vi "Control - PID Control.vi"() -> ()   [LabVIEW 2013, in "PID Control Workspace Object.lvlib"]
doc: "Sample numeric display item."
uses:
  PID Control Workspace Object.lvlib
  <vilib>/NI Veristand/Display Template Support/Display Template Support.llb/cluster_Screen Item Settings.ctl
  <vilib>/NI Veristand/Display Template Support/Display Template Support.llb/cluster_Graph Scale Settings.ctl
  <vilib>/NI Veristand/Display Template Support/Display Template Support.llb/cluster_Graph Plot Settings.ctl
  NationalInstruments.VeriStand.SystemStorage
  <vilib>/NI Veristand/Display Template Support/Display Template Support.llb/enum_Display Template Handler Minimal To Widget Msg.ctl
  <vilib>/NI Veristand/Display Template Support/Display Template Support.llb/enum_Display Template Handler Minimal To Workspace.ctl
  Shared/Types/Workspace Object Cached Settings.ctl
  Shared/Types/Workspace Object State Variables.ctl
  <vilib>/NI Veristand/Execution/Workspace/UDPChannelStreamSession.ctl
  Shared/Types/UDP Streaming Command Cluster.ctl
  Shared/Types/UDP Streaming State.ctl
  NationalInstruments.VeriStand.ClientAPI
  <vilib>/NI Veristand/Execution/Workspace/UDP Stream Packet.ctl
  <vilib>/NI Veristand/Display Template Support/Display Template Support.llb/sub_Display Template Handler Custom.vi
  Shared/Constants.vi
  <vilib>/NI Veristand/Execution/Workspace/NI VeriStand - Set Single Channel Value.vi
  <vilib>/NI Veristand/Execution/Workspace/NI VeriStand - Get Multiple Channel Values.vi
  <vilib>/Utility/tcp.llb/UDP Multicast Read-Only Open.vi
  Shared/Control Addon Shared.lvlib
  <vilib>/NI Veristand/Execution/Workspace/NI_VS Workspace ExecutionAPI.lvlib
panel:
  in  "Revert":bool
  in  "Apply":bool
  in  "Manual Output":dbl
  in  "Manual Control":bool
  in  "Setpoint":dbl
  in  "NIVS.System Definition Root":refnum<k24>
  in  "NIVS.Gateway IP Address":string
  in  "Hold":bool
  in  "Autoscale Y":bool=TRUE
  in  "Autoscale X":bool=TRUE
  out "Chart":waveform(dbl)[](graph)
  out "Control Name":string
  in  "Item.Data":T1
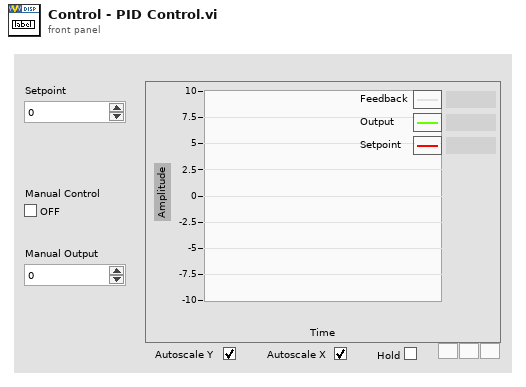
[diagram p1: front panel]
types:
  T1 = typedef "cluster_Screen Item Settings.ctl" = cluster{"Template VI":string, "Position X":i32, "Position Y":i32, "Custom":string, "Show Title Bar":bool, "ID":i32, "Always On Top":bool, "Allow Resize":bool, "Allow Minimize":bool, "Allow Close":bool, "Size to Screen":bool, "Screen.ID":i32, "State":enum16{"Normal", "New"}, "Title":string, "Window Bounds":cluster{"[0]":i16, "[1]":i16, "[2]":i16, "[3]":i16}, "Channel Ref":u64, "Unit":string, "Default Units?":bool, "Flash Limit?":bool, "Color 1":u32, "Color 2":u32, "Color 3":u32, "Color 4":u32, "Bck Color":u32, "Fore Color":u32, "Limit 1":dbl, "Limit 2":dbl, "Limit 3":dbl, "Limit 4":dbl, "Limit Mode 1":i32, "Limit Mode 2":i32, "Limit Mode 3":i32, "Limit Mode 4":i32, "Scale Precision":i32, "Scale Min":dbl, "Scale Max":dbl, "Format":i32, "Precision":i32, "Background Type":i32, "IDs":i32[], "Units":string[], "Labels":string[], "Scale Factor":dbl, "Scale Offset":dbl, "YScale Index":u32[], "XScale":T2, "YScales":T2[], "Plots":T3[], "Update Period":dbl, "History Length":dbl, "My.Ref":refnum<vi>, "Is Control?":bool, "Channel Paths":string[], "Custom Data":variant}
  T2 = typedef "cluster_Graph Scale Settings.ctl" = cluster{"Format":u8, "Precision":u8, "Fit":u8, "Label":string, "Use Default Label":bool, "Label Visible":bool, "Min":dbl, "Max":dbl}
  T3 = typedef "cluster_Graph Plot Settings.ctl" = cluster{"Bar Style":u8, "Fill To":i16, "Fill/PtColor":u32, "Line Style":u8, "Line Width":u8, "Color":u32, "Interp":u8, "Point Style":u8}
  T4 = typedef "Control Addon Shared.lvlib/UDP Streaming State.ctl" = enum8{"Idle", "Start Acq", "Run", "Stop Acq", "Exit"}
  T5 = typedef "Control Addon Shared.lvlib/UDP Streaming Command Cluster.ctl" = cluster{"Action":T4, "Channels":string[]}
  T6 = typedef "NI_VS Workspace ExecutionAPI.lvlib/UDPChannelStreamSession.ctl" = refnum<k24>
  T7 = cluster{"Initialized Waveform":waveform(dbl)[], "VS UDP Session":T6, "Channel IDs":i32[], "Packet IDs":i32[], "Max Packet Size":i32, "UDP Ref":refnum<k16>}
  T8 = typedef "Control Addon Shared.lvlib/Workspace Object State Variables.ctl" = cluster{"Cached":T9, "Found?":bool, "UDP Channels":string[], "Connected?":bool, "Previous Values":dbl[], "Slow Channels":string[], "Pending Change?":bool}
  T9 = typedef "Control Addon Shared.lvlib/Workspace Object Cached Settings.ctl" = cluster{"Path":string}
  T10 = typedef "enum_Display Template Handler Minimal To Workspace.ctl" = cluster{"Operation":enum16{"SetCustomData", "DeleteItem"}, "Data":variant}
  T11 = typedef "enum_Display Template Handler Minimal To Widget Msg.ctl" = enum16{"Stop", "LaunchConfigDialog"}
  T12 = typedef "NI_VS Workspace ExecutionAPI.lvlib/WorkspaceAPI.ctl" = refnum<k24>
  T13 = typedef "NI_VS Workspace ExecutionAPI.lvlib/SystemStateEventRef.ctl" = cluster{"CustDatRef":refnum<user-event>, "EvtRef":refnum<k27>}
  T14 = typedef "NI_VS Workspace ExecutionAPI.lvlib/SystemStateRegEventRef.ctl" = refnum<event-registration>
  T15 = cluster{"Event Registration Refnum":refnum<event-registration>, "SystemChangeEventRef":T14}
  T16 = typedef "NI_VS Workspace ExecutionAPI.lvlib/SystemState.ctl" = u8
  T17 = typedef "NI_VS Workspace ExecutionAPI.lvlib/UDP Stream Packet.ctl" = cluster{"ID":i32, "t0":dbl, "dt":dbl, "Channel IDs":i32[], "Channel Data":dbl[][], "Sample Offset":u64}
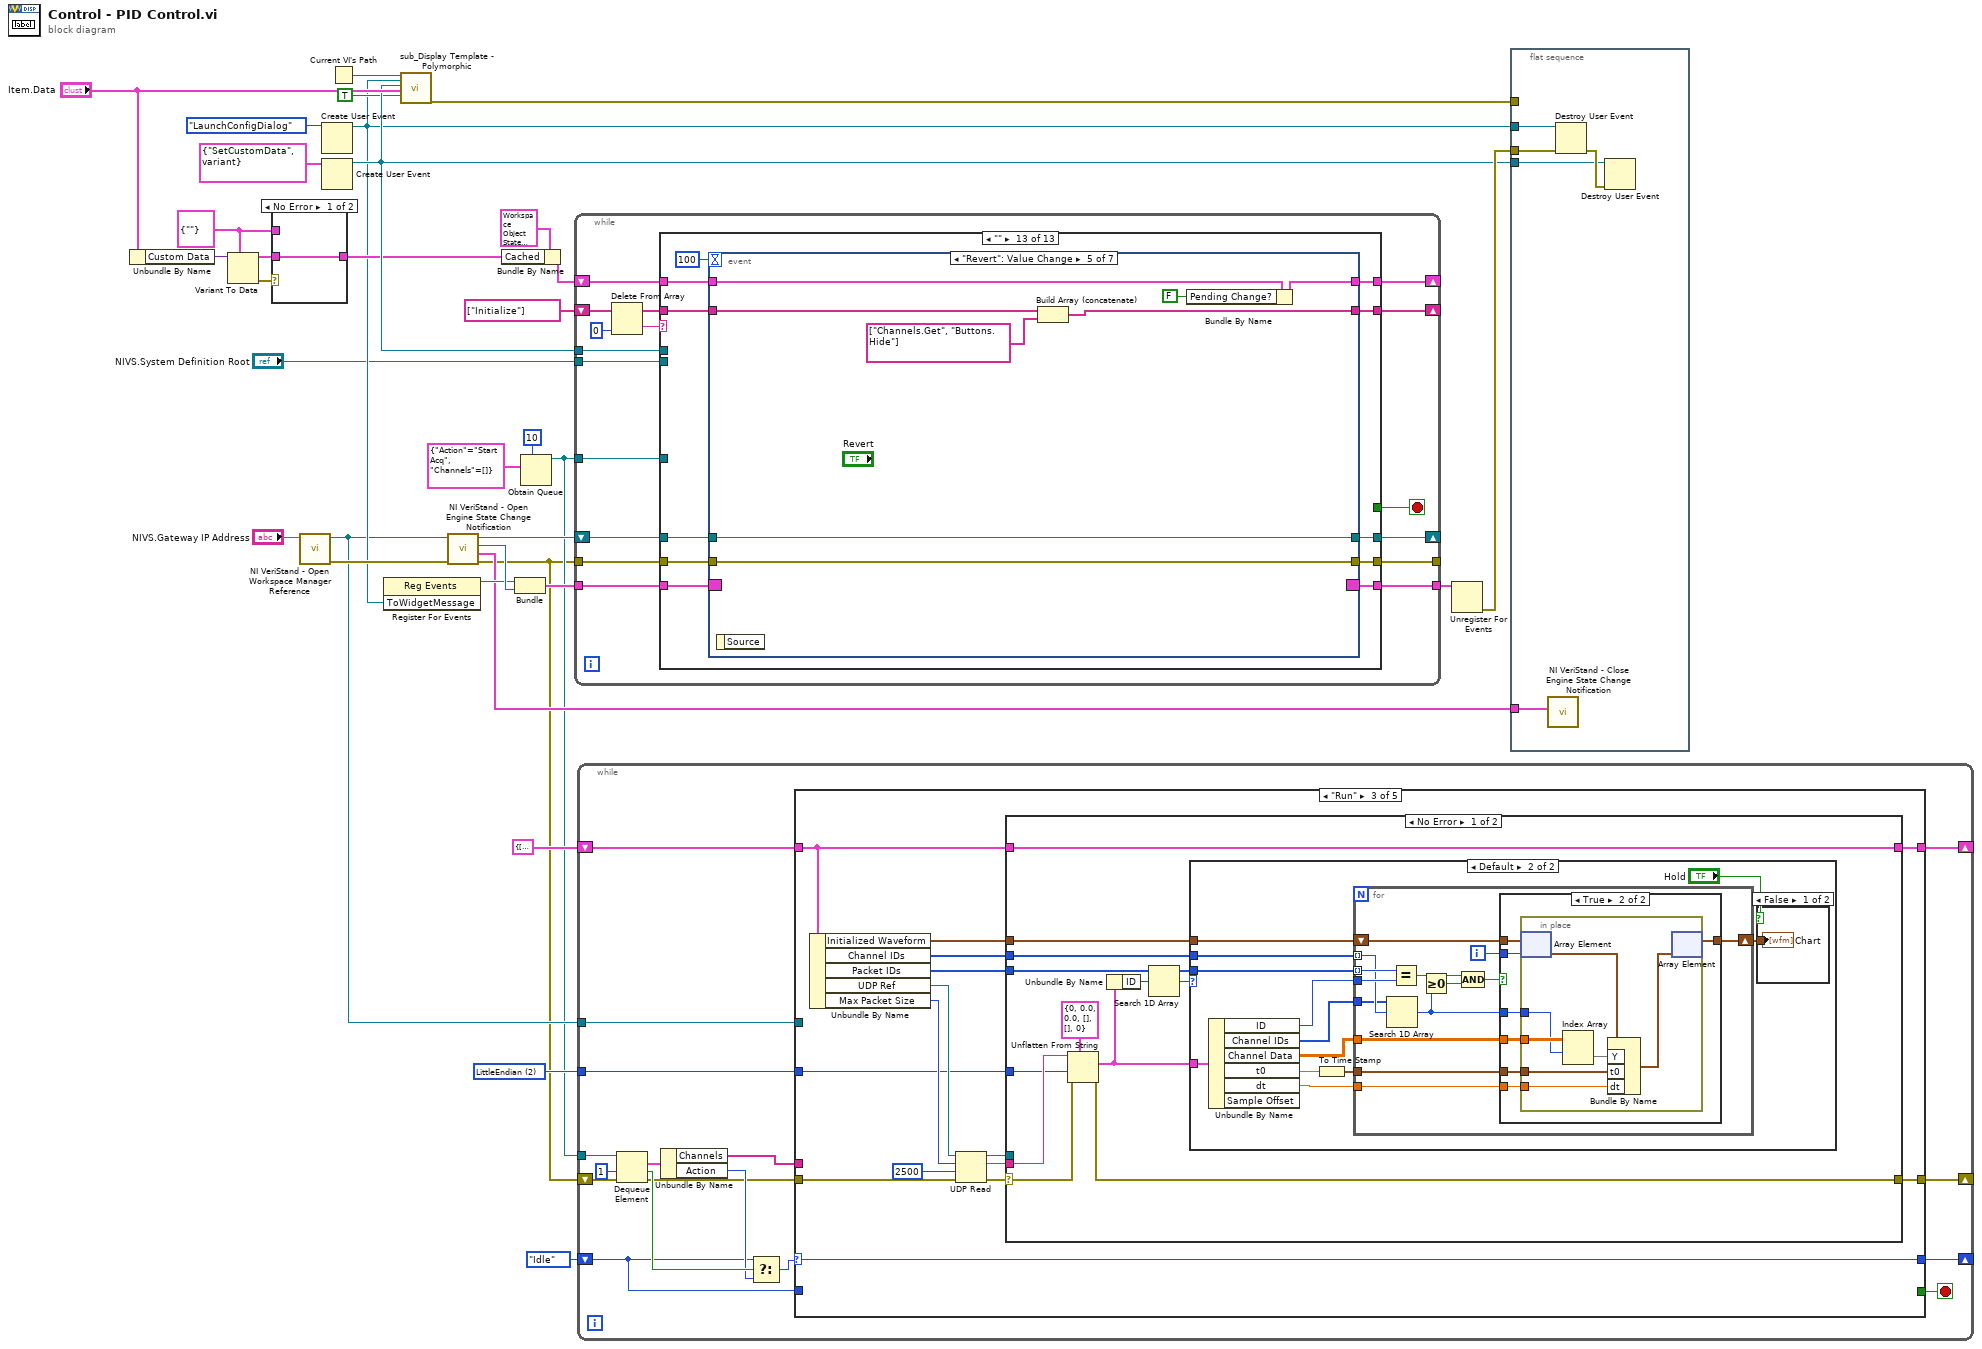
[diagram p0: block diagram]
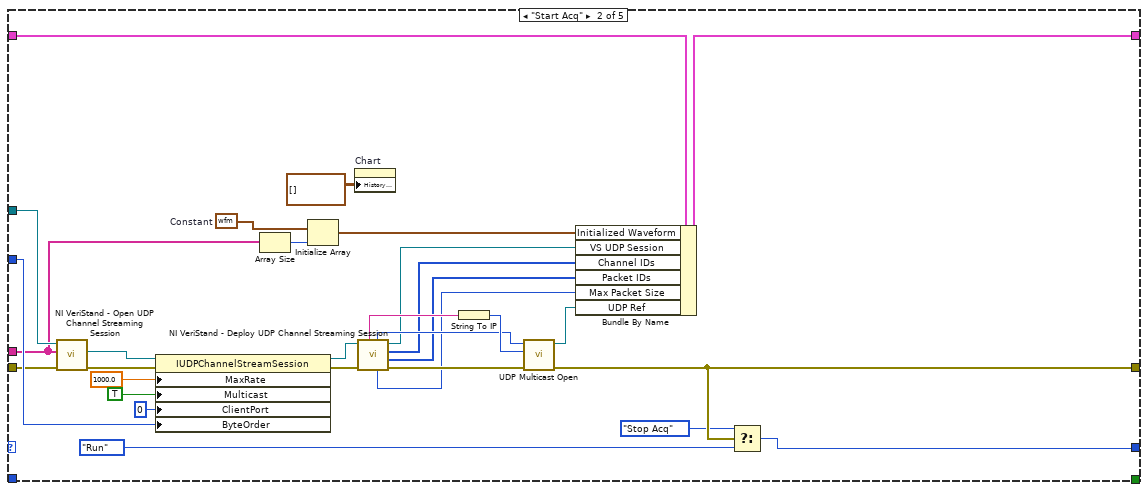
[diagram p3: hidden frame]
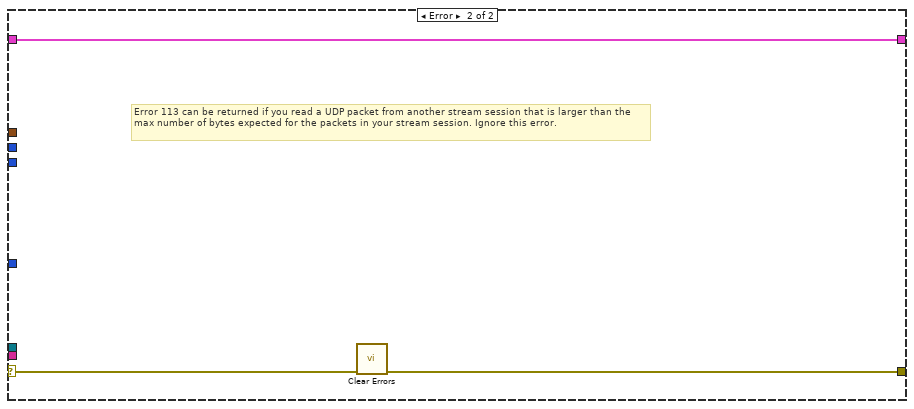
[diagram p7: hidden frame]
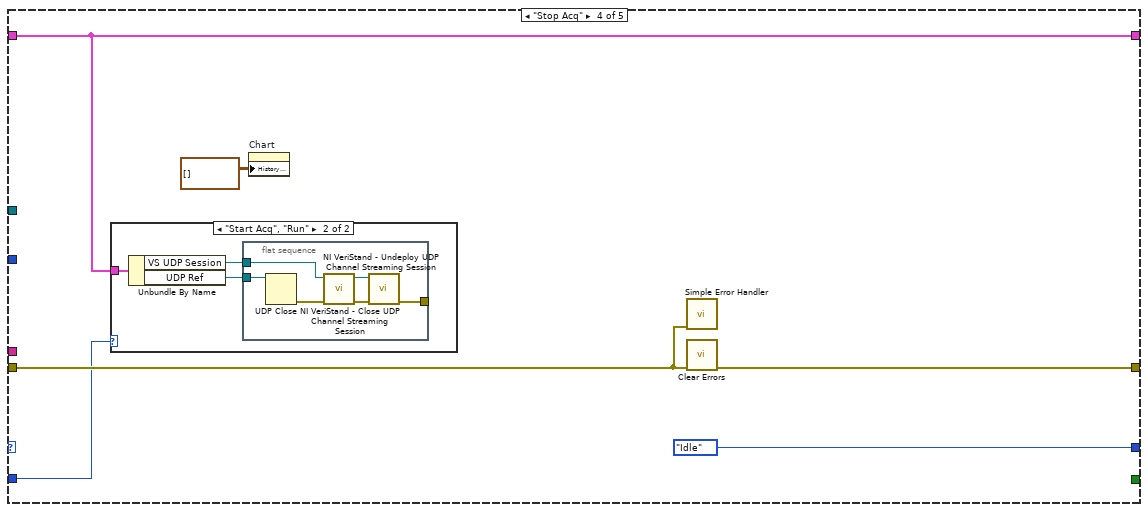
[diagram p8: hidden frame]
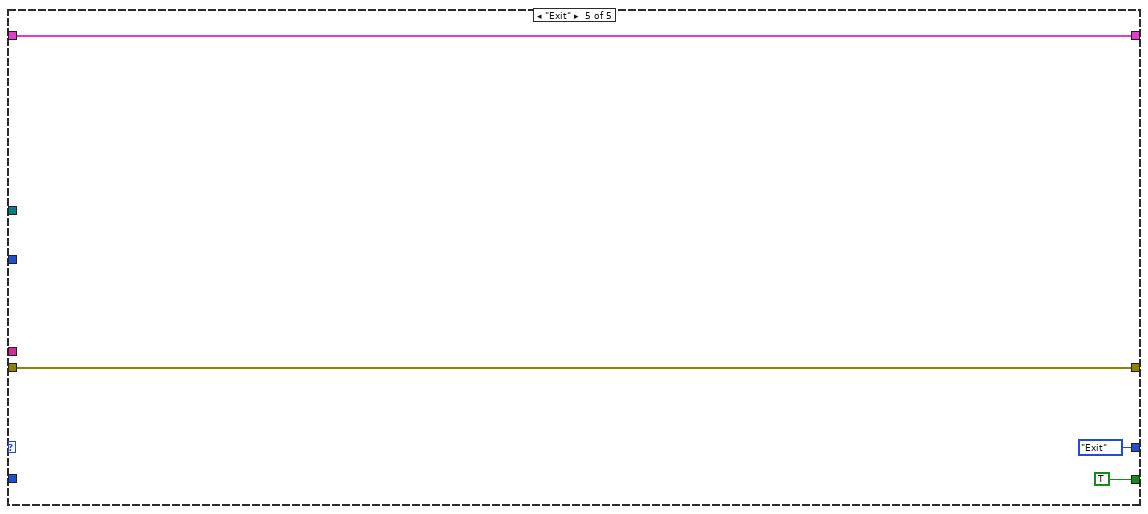
[diagram p10: hidden frame]
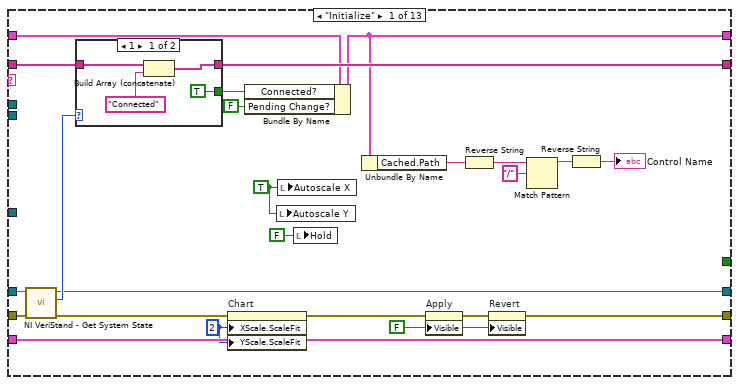
[diagram p12: hidden frame]
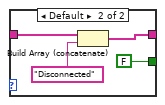
[diagram p13: hidden frame]
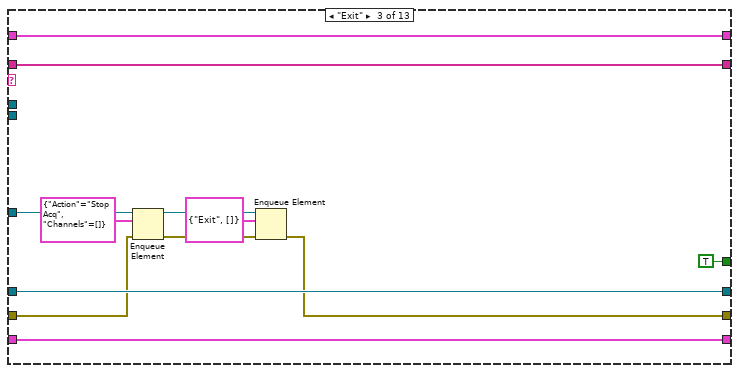
[diagram p15: hidden frame]
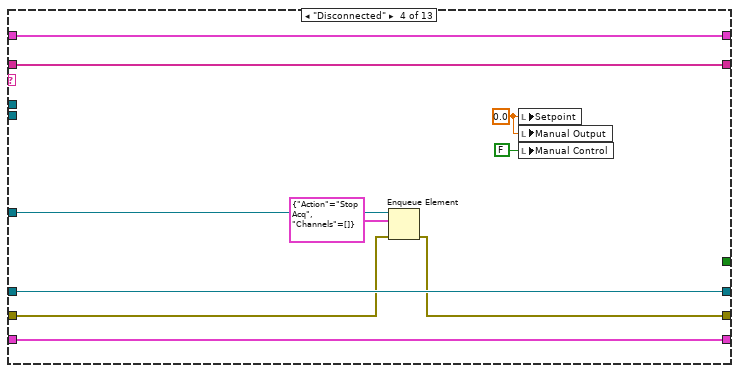
[diagram p16: hidden frame]
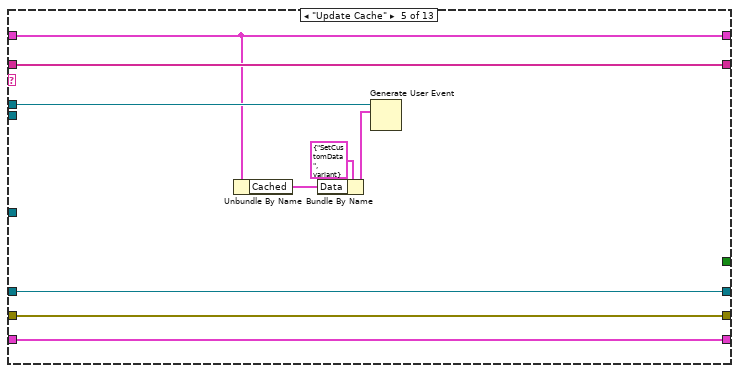
[diagram p17: hidden frame]
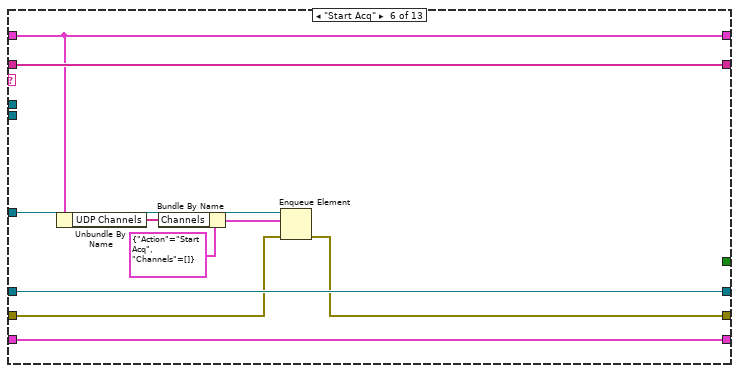
[diagram p18: hidden frame]
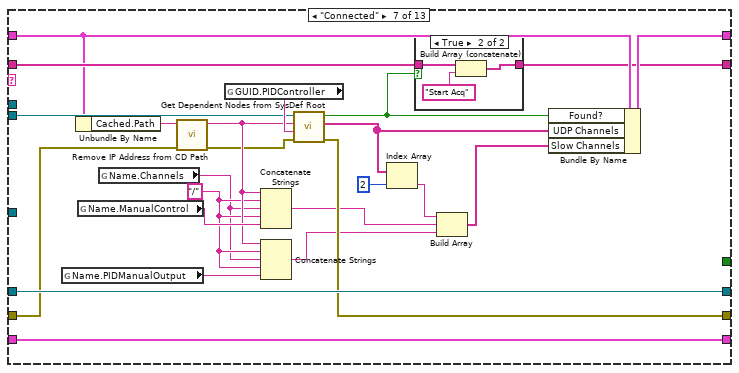
[diagram p19: hidden frame]
diagram:
  w6 = 2 items=["BigEndian", "NativeHostOrder", "LittleEndian"] ("Byte Order")
  w14 = T9 {"Path"=""}
  n1 = Unbundle By Name("Item.Data") -> ("Custom Data"=w18:variant)
  n2 = Variant To Data(type=w14, Variant=w18) -> (data=w15:T9, error out=w16:errorcluster)  [unwired: 1 in]
  n3 = case shown="No Error" w16 {
    tunnel: w15 -> [w35 _]
    tunnel: [w35 w36] -> w11
    tunnel: w14 -> [_ w36]
    frame No Error {
    }
    frame Error {
    }
  }
  n4 = call <vilib>:"NI VeriStand - Open Workspace Manager Reference.vi"("Gateway IP Address (\"\": localhost)"="NIVS.Gateway IP Address") -> ("error out"=w25:errorcluster, "WorkspaceManager"=w8:T12)  [unwired: 9 in]
  n5 = Create User Event(user event datatype=enum_Display_Template_Handler_Minimal_To_Widget_Msg."LaunchConfigDialog" ("ToWidgetMessage")) -> (user event=w10:refnum<user-event>)  [unwired: 1 in, 1 out]
  n6 = Create User Event(user event datatype=T10 {"Operation"=enum."SetCustomData", "Data"=variant} ("Data")) -> (user event=w28:refnum<user-event>)  [unwired: 1 in, 1 out]
  n7 = Current VI's Path() -> (path=w30:path)
  n8 = register-events(w10) -> (reference out=w23:refnum<event-registration>)  [unwired: 2 in, 1 out]
  n9 = call-poly <vilib>:"sub_Display Template - Polymorphic.vi"("Parent.Path"=w30, "ToWidgetEvent"=w10, "ToWorkspace"=w28, "Item.Data"="Item.Data", "Resizable"=TRUE) -> ("error out"=w34:errorcluster)  [unwired: 1 in, 13 out]
  n10 = call <vilib>:"NI VeriStand - Open Engine State Change Notification.vi"("error in (no error)"=w25, "WorkspaceManager in"=w8) -> ("error out"=w1:errorcluster, "SystemStateRefs"=w21:T13, "SystemChangeEventRef"=w24:T14, "WorkspaceManager out"=w19:T12)  [unwired: 6 in]
  n11 = Bundle By Name(cluster=T8 {"Cached"={"Path"=""}, "Found?"=FALSE, "UDP Channels"=[], "Connected?"=FALSE, "Previous Values"=[0.0, 0.0, 0.0], "Slow Channels"=[], "Pending Change?"=FALSE}, "Cached"=w11) -> (w12:T8)
  n12 = Bundle("Event Registration Refnum"=w23, "SystemChangeEventRef"=w24) -> (w22:T15)  [unwired: 1 in]
  n13 = Obtain Queue(max queue size (-1, unlimited)=10, element data type=T5 {"Action"=enum."Start Acq", "Channels"=[]}) -> (queue out=w3:refnum<queue>)  [unwired: 3 in, 2 out]
  n14 = while {
    tunnel: w22 -> [w53]
    tunnel: w28 -> [w51]
    shift-right: [w45] -> _
    shift-left: string[] ["Initialize"] -> [w49]
    shift-right: [w43] -> _
    shift-left: w19 -> [w42]
    tunnel: w1 -> [w47]
    tunnel: [w44] -> w17
    tunnel: [w40] -> _
    shift-right: [w39] -> _
    shift-left: w12 -> [w41]
    tunnel: "NIVS.System Definition Root" -> [w38]
    tunnel: w3 -> [w37]
    stop <- w52 stop-if-true
    n15 = Delete From Array(array=w49, index=0) -> (deleted portion=w48:string, array with subset deleted=w46:string[])  [unwired: 1 in]
    n16 = case shown="\"\"" w48 {
      tunnel: w53 -> [w71 w89 w101 w111 w120 w130 w154 w171 w198 w230 w238 w256 w277]
      tunnel: [_ _ TRUE _ _ _ _ _ _ _ _ _ _] -> w52
      tunnel: [w73 w90 w102 w112 w121 w131 w137 w161 w199 w231 w239 w257 w274] -> w45
      tunnel: w51 -> [_ _ _ _ w117 _ _ _ _ _ _ _ _]
      tunnel: w47 -> [w76 w87 w93 w107 w118 w123 w141 w169 w186 w225 w233 w244 w270]
      tunnel: w46 -> [w74 w90 w102 w112 w121 w131 w155 w160 w199 w231 w239 w257 w273]
      tunnel: [w71 w89 w101 w111 w120 w130 w154 w171 w198 w230 w238 w256 w275] -> w44
      tunnel: [w72 w88 w100 w110 w119 w129 w153 w170 w183 w229 w237 w242 w271] -> w43
      tunnel: w42 -> [w75 w88 w100 w110 w119 w129 w153 w170 w184 w229 w237 w245 w272]
      tunnel: w41 -> [w65 w86 w99 w109 w114 w128 w149 w165 w182 w228 w236 w240 w267]
      tunnel: [w55 w87 w92 w106 w118 w122 w152 w169 w185 w224 w232 w243 w269] -> w40
      tunnel: [w64 w86 w99 w109 w114 w128 w148 w164 w181 w228 w236 w241 w268] -> w39
      tunnel: w38 -> [_ _ _ _ _ _ w150 w167 _ _ _ _ _]
      tunnel: w37 -> [_ _ w98 w108 _ w127 _ _ _ _ _ _ _]
      frame "Initialize" {
        w54 = FALSE ("Hold")
        w61 = u8 2 ("X Scale.Scale Fit")
        w62 = TRUE ("Autoscale X")
        n17 = call <vilib>:"NI VeriStand - Get System State.vi"("error in (no error)"=w76, "WorkspaceManager in"=w75) -> ("error out"=w60:errorcluster, "System State"=w77:T16, "WorkspaceManager  out"=w72:T12)  [unwired: 5 in, 2 out]
        n18 = case shown="1" w77 {
          tunnel: w74 -> [w81 w85]
          tunnel: [w80 w84] -> w73
          tunnel: [TRUE FALSE] -> w63
          frame 1 {
            n19 = Build Array (concatenate)(w81, "Connected") -> (w80:string[])
          }
          frame Default {
            n20 = Build Array (concatenate)(w85, "Disconnected") -> (w84:string[])
          }
        }
        n21 = property on="Chart" class="WFChart (strict)"(error in=w60, "XScale.ScaleFit"=w61, "YScale.ScaleFit"=w61) -> (error out=w57:errorcluster)  [unwired: 1 in, 1 out]
        n22 = Bundle By Name(cluster=w65, "Connected?"=w63, "Pending Change?"=FALSE) -> (w64:T8)
        n23 = local write "Autoscale Y"(w62) -> ()
        n24 = local write "Autoscale X"(w62) -> ()
        n25 = local write "Hold"(FALSE ("Hold")) -> ()
        n26 = Unbundle By Name(w64) -> ("Cached.Path"=w67:string)
        n27 = property on="Apply" class="Bool"(error in=w57, "Visible"=w54) -> (error out=w56:errorcluster)  [unwired: 1 in, 1 out]
        n28 = Reverse String(1:w67) -> (0:w70:string)
        n29 = property on="Revert" class="Bool"(error in=w56, "Visible"=w54) -> (error out=w55:errorcluster)  [unwired: 1 in, 1 out]
        n30 = Match Pattern(string=w70, regular expression="/") -> (before substring=w66:string)  [unwired: 1 in, 3 out]
        n31 = Reverse String(1:w66) -> (0:→"Control Name":string)
      }
      frame Default {
      }
      frame "Exit" {
        n32 = Enqueue Element(queue=w98, element=T5 {"Action"=enum."Stop Acq", "Channels"=[]}, error in (no error)=w93) -> (queue out=w96:refnum<queue>, error out=w94:errorcluster)  [unwired: 1 in, 1 out]
        n33 = Enqueue Element(queue=w96, element=T5 {"Action"=enum."Exit", "Channels"=[]}, error in (no error)=w94) -> (error out=w92:errorcluster)  [unwired: 1 in, 2 out]
      }
      frame "Disconnected" {
        w104 = 0.0 ("Setpoint")
        n34 = Enqueue Element(queue=w108, element=T5 {"Action"=enum."Stop Acq", "Channels"=[]}, error in (no error)=w107) -> (error out=w106:errorcluster)  [unwired: 1 in, 2 out]
        n35 = local write "Setpoint"(w104) -> ()
        n36 = local write "Manual Output"(w104) -> ()
        n37 = local write "Manual Control"(FALSE ("Manual Control")) -> ()
      }
      frame "Update Cache" {
        n38 = Unbundle By Name(w114) -> ("Cached"=w113:T9)
        n39 = Bundle By Name(cluster=T10 {"Operation"=enum."SetCustomData", "Data"=variant} ("event data"), "Data"=w113) -> (w115:T10)
        n40 = Generate User Event(user event=w117, event data cluster=w115) -> ()  [unwired: 2 in, 2 out]
      }
      frame "Start Acq" {
        n41 = Unbundle By Name(w128) -> ("UDP Channels"=w125:string[])
        n42 = Bundle By Name(cluster=T5 {"Action"=enum."Start Acq", "Channels"=[]}, "Channels"=w125) -> (w124:T5)
        n43 = Enqueue Element(queue=w127, element=w124, error in (no error)=w123) -> (error out=w122:errorcluster)  [unwired: 1 in, 2 out]
      }
      frame "Connected" {
        w134 = "/" ("string")
        n44 = global read "Constants.vi" "Name.PIDManualOutput"() -> (w144:string)
        n45 = Unbundle By Name(w149) -> ("Cached.Path"=w147:string)
        n46 = global read "Constants.vi" "Name.ManualControl"() -> (w146:string)
        n47 = global read "Constants.vi" "Name.Channels"() -> (w133:string)
        n48 = call "Remove IP Address from CD Path.vi"("error in (no error)"=w141, "CD Path"=w147) -> ("error out"=w140:errorcluster, "Path"=w145:string)  [unwired: 8 in]
        n49 = global read "Constants.vi" "GUID.PIDController"() -> (w151:string)
        n50 = Concatenate Strings(w145, w134, w133, w134, w146) -> (w143:string)
        n51 = Concatenate Strings(w145, w134, w133, w134, w144) -> (w142:string)
        n52 = call "Get Dependent Nodes from SysDef Root.vi"("error in (no error)"=w140, "GUID"=w151, "Path"=w145, "SysDef Ref"=w150) -> ("error out"=w152:errorcluster, "Channels"=w136:string[], "Found"=w132:bool)  [unwired: 5 in]
        n53 = Index Array(array=w136, index=2) -> (element=w138:string)
        n54 = case shown="True" w132 {
          tunnel: w155 -> [w156 w159]
          tunnel: [w156 w158] -> w137
          frame False {
          }
          frame True {
            n55 = Build Array (concatenate)(w159, "Start Acq") -> (w158:string[])
          }
        }
        n56 = Build Array(w138, w143, w142) -> (w135:string[])
        n57 = Bundle By Name(cluster=w149, "Found?"=w132, "UDP Channels"=w136, "Slow Channels"=w135) -> (w148:T8)
      }
      frame "Configure" {
        n58 = Unbundle By Name(w165) -> ("Cached.Path"=w166:string)
        n59 = call "Select Controller.vi"("Type"=enum16{"PID", "Industrial"}."PID", "CD Path"=w166, "NIVS.System Definition Root"=w167) -> ("Cancelled?"=w163:bool, "Custom Device Path Out"=w162:string)  [unwired: 6 in, 1 out]
        n60 = case shown="False" w163 {
          tunnel: w165 -> [w177 w178]
          tunnel: [w176 w178] -> w164
          tunnel: w162 -> [w175 _]
          tunnel: [w173 w179] -> w161
          tunnel: w160 -> [w174 w179]
          frame False {
            n61 = Bundle By Name(cluster=w177, "Cached.Path"=w175) -> (w176:T8)
            n62 = Build Array (concatenate)(w174, string[] ["Update Cache", "Initialize"]) -> (w173:string[])
          }
          frame True {
          }
        }
      }
      frame "Channels.Set" {
        n63 = Unbundle By Name(w182) -> ("Found?"=w189:bool, "Connected?"=w192:bool, "Previous Values"=w191:dbl[], "Slow Channels"=w193:string[])
        n64 = Boolean To (0,1)(Boolean="Manual Control") -> (0, 1=w188:i16)
        n65 = Build Array("Setpoint", w188, "Manual Output") -> (w194:dbl[])
        n66 = Not Equal?(x=w191, y=w194) -> (x != y?=w197:bool[])
        n67 = Compound Arithmetic op=AND(w189, w192) -> (w190:bool)
        n68 = case shown="True" w190 {
          tunnel: w197 -> [_ w208]
          tunnel: w194 -> [_ w207]
          tunnel: w186 -> [w201 w206]
          tunnel: [w201 w205] -> w185
          tunnel: w184 -> [w200 w204]
          tunnel: [w200 w203] -> w183
          tunnel: w193 -> [_ w202]
          frame False {
          }
          frame True {
            n69 = for {
              shift-right: [w214] -> w205
              shift-left: w206 -> [w215]
              shift-right: [w213] -> w203
              shift-left: w204 -> [w212]
              tunnel: w208 -> [w211] mode=indexing
              tunnel: w207 -> [w210] mode=indexing
              tunnel: w202 -> [w209] mode=indexing
              n70 = case shown="True" w211 {
                tunnel: w215 -> [w217 w223]
                tunnel: [w217 w222] -> w214
                tunnel: [w216 w221] -> w213
                tunnel: w212 -> [w216 w220]
                tunnel: w210 -> [_ w219]
                tunnel: w209 -> [_ w218]
                frame False {
                }
                frame True {
                  n71 = call-poly <vilib>:"NI VeriStand - Set Channel Value.vi"("error in (no error)"=w223, "Value"=w219, "Channel"=w218, "WorkspaceManager in"=w220) -> ("error out"=w222:errorcluster, "WorkspaceManager out"=w221:T12)  [unwired: 6 in]
                }
              }
            }
          }
        }
        n72 = Bundle By Name(cluster=w182, "Pending Change?"=FALSE) -> (w181:T8)
      }
      frame "Buttons.Hide" {
        w226 = FALSE ("Hold")
        n73 = property on="Apply" class="Bool"(error in=w225, "Visible"=w226) -> (error out=w227:errorcluster)  [unwired: 1 in, 1 out]
        n74 = property on="Revert" class="Bool"(error in=w227, "Visible"=w226) -> (error out=w224:errorcluster)  [unwired: 1 in, 1 out]
      }
      frame "Buttons.Show" {
        w234 = TRUE ("Hold")
        n75 = property on="Apply" class="Bool"(error in=w233, "Visible"=w234) -> (error out=w235:errorcluster)  [unwired: 1 in, 1 out]
        n76 = property on="Revert" class="Bool"(error in=w235, "Visible"=w234) -> (error out=w232:errorcluster)  [unwired: 1 in, 1 out]
      }
      frame "Channels.Get" {
        n77 = Unbundle By Name(w240) -> ("Found?"=w248:bool, "Connected?"=w254:bool, "Slow Channels"=w255:string[])
        n78 = Compound Arithmetic op=AND(w248, w254) -> (w249:bool)
        n79 = case shown="False" w249 {
          tunnel: w244 -> [w260 w266]
          tunnel: [w260 w265] -> w243
          tunnel: w245 -> [w259 w264]
          tunnel: [w259 w263] -> w242
          tunnel: w255 -> [_ w262]
          tunnel: [dbl[] [0.0, 0.0, 0.0] ("Values") w261] -> w253
          frame False {
          }
          frame True {
            n80 = call-poly <vilib>:"NI VeriStand - Get Channel Value.vi"("error in (no error)"=w266, "Channels"=w262, "WorkspaceManager in"=w264) -> ("error out"=w265:errorcluster, "Values"=w261:dbl[], "WorkspaceManager out"=w263:T12)  [unwired: 6 in]
          }
        }
        n81 = Index Array(array=w253) -> (element #1=w252:dbl, element #2=w247:dbl, element #3=w246:dbl)  [unwired: 3 in]
        n82 = To Long Integer(number=w247) -> (32bit integer=w251:i32)
        n83 = Not Equal To 0?(x=w251) -> (x != 0?=w250:bool)
        n84 = local write "Setpoint"(w252) -> ()
        n85 = local write "Manual Control"(w250) -> ()
        n86 = local write "Manual Output"(w246) -> ()
        n87 = Bundle By Name(cluster=w240, "Previous Values"=w253) -> (w241:T8)
      }
      frame "" {
        n88 = event shown="[4] \"Revert\": Value Change" {
          selector: w277 -> [_ _ _ _ _ _ _]
          dyn-events: [_ _ _ _ _ _ _] -> w275
          timeout: 100 -> [_ _ _ _ _ _ _]
          tunnel: [w280 w300 w301 w309 w318 w327 w347] -> w274
          tunnel: w273 -> [w281 w300 w303 w310 w319 w328 w346]
          tunnel: w272 -> [w282 w299 w307 w314 w322 w331 w348]
          tunnel: [w282 w299 w307 w314 w322 w330 w348] -> w271
          tunnel: w270 -> [w283 w293 w308 w313 w321 w333 w345]
          tunnel: [w283 w292 w308 w313 w321 w332 w345] -> w269
          tunnel: [w279 w298 w304 w312 w316 w325 w344] -> w268
          tunnel: w267 -> [w279 w298 w305 w312 w317 w326 w344]
          event Timeout {
            n89 = event-data() -> ()  [unwired: 2 out]
            n90 = Unbundle By Name(w279) -> ("Pending Change?"=w278:bool)
            n91 = case shown="False" w278 {
              tunnel: w281 -> [w285 w287]
              tunnel: [w284 w287] -> w280
              frame False {
                n92 = Build Array (concatenate)(w285, "Channels.Get") -> (w284:string[])
              }
              frame True {
              }
            }
          }
          event "Autoscale Y", "Autoscale X": Value Change {
            n93 = event-data() -> ()  [unwired: 2 out]
            n94 = Select(t=u8 2, s="Autoscale X", f=u8 0 ("X Scale.Scale Fit")) -> (s? t:f=w295:u8)
            n95 = Select(t=u8 2, s="Autoscale Y", f=u8 0 ("X Scale.Scale Fit")) -> (s? t:f=w288:u8)
            n96 = property on="Chart" class="WFChart (strict)"(error in=w293, "XScale.ScaleFit"=w295, "YScale.ScaleFit"=w288) -> (error out=w292:errorcluster)  [unwired: 1 in, 1 out]
          }
          event "Setpoint", "Manual Control", "Manual Output": Value Change {
            n97 = event-data() -> ()  [unwired: 2 out]
            n98 = Bundle By Name(cluster=w305, "Pending Change?"=TRUE) -> (w304:T8)
            n99 = Build Array (concatenate)(w303, "Buttons.Show") -> (w301:string[])
          }
          event "Apply": Value Change {
            n100 = event-data() -> ()  [unwired: 2 out]
            n101 = Build Array (concatenate)(w310, string[] ["Channels.Set", "Buttons.Hide"]) -> (w309:string[])
          }
          event "Revert": Value Change {
            n102 = event-data() -> ()  [unwired: 2 out]
            n103 = Build Array (concatenate)(w319, string[] ["Channels.Get", "Buttons.Hide"]) -> (w318:string[])
            n104 = Bundle By Name(cluster=w317, "Pending Change?"=FALSE) -> (w316:T8)
          }
          event User Event {
            n105 = event-data() -> ()  [unwired: 2 out]
            n106 = call <vilib>:"NI VeriStand - Get System State.vi"("error in (no error)"=w333, "WorkspaceManager in"=w331) -> ("error out"=w332:errorcluster, "System State"=w329:T16, "WorkspaceManager  out"=w330:T12)  [unwired: 5 in, 2 out]
            n107 = case shown="Default" w329 {
              tunnel: w328 -> [w338 w343]
              tunnel: [w337 w342] -> w327
              tunnel: [w335 w340] -> w324
              tunnel: w326 -> [w335 w340]
              tunnel: [TRUE FALSE] -> w323
              frame 1 {
                n108 = Build Array (concatenate)(w338, "Connected") -> (w337:string[])
              }
              frame Default {
                n109 = Build Array (concatenate)(w343, "Disconnected") -> (w342:string[])
              }
            }
            n110 = Bundle By Name(cluster=w324, "Connected?"=w323) -> (w325:T8)
          }
          event User Event {
            n111 = event-data() -> ("ToWidgetMessage"=w349:T11)  [unwired: 1 out]
            n112 = case shown="\"Stop\"" w349 {
              tunnel: [w350 w352 w355] -> w347
              tunnel: w346 -> [w350 w353 w356]
              frame Default {
              }
              frame "Stop" {
                n113 = Build Array (concatenate)(w353, "Exit") -> (w352:string[])
              }
              frame "LaunchConfigDialog" {
                n114 = Build Array (concatenate)(w356, "Configure") -> (w355:string[])
              }
            }
          }
        }
      }
    }
  }
  n115 = while {
    tunnel: w8 -> [w373]
    tunnel: w6 -> [w371]
    tunnel: w3 -> [w370]
    shift-right: [w364] -> _
    shift-left: UDP_Streaming_State."Idle" ("Action") -> [w357]
    shift-right: [w363] -> _
    shift-left: T7 {"Initialized Waveform"=[], "VS UDP Session"=refnum, "Channel IDs"=[], "Packet IDs"=[], "Max Packet Size"=0, "UDP Ref"=refnum} -> [w372]
    shift-right: [w360] -> _
    shift-left: w1 -> [w359]
    stop <- w362 stop-if-true
    n116 = Dequeue Element(queue=w370, timeout in ms (-1)=1, error in (no error)=w359) -> (element=w369:T5, timed out?=w367:bool, error out=w361:errorcluster)  [unwired: 1 out]
    n117 = Unbundle By Name(w369) -> ("Channels"=w358:string[], "Action"=w366:T4)
    n118 = Select(t=w357, s=w367, f=w366) -> (s? t:f=w365:T4)
    n119 = case shown="\"Run\"" w365 {
      selector: w365 -> [w374 _ w410 _ _]
      tunnel: w373 -> [_ w394 _ _ _]
      tunnel: w372 -> [w376 w393 w411 w484 w495]
      tunnel: w371 -> [_ w386 w407 _ _]
      tunnel: [w376 w385 w412 w484 w495] -> w363
      tunnel: [w374 w380 w410 UDP_Streaming_State."Idle" ("Action") UDP_Streaming_State."Exit" ("Action")] -> w364
      tunnel: [_ _ _ _ TRUE] -> w362
      tunnel: w361 -> [w375 w384 w409 w482 w494]
      tunnel: [w375 w383 w408 w481 w494] -> w360
      tunnel: w358 -> [_ w378 _ _ _]
      tunnel: w357 -> [_ _ _ w480 _]
      frame "Idle" {
      }
      frame "Start Acq" {
        w400 = waveform(dbl) {"t0"=timestamp(0 s since 1904-01-01), "dt"=1.0, "Y"=[]}  # Constant
        n120 = call <vilib>:"NI VeriStand - Open UDP Channel Streaming Session.vi"("error in (no error)"=w384, "Channels"=w378, "WorkspaceManager in"=w394) -> ("error out"=w404:errorcluster, "UDPChannelStreamSession out"=w401:T6)  [unwired: 6 in, 1 out]
        n121 = property class="IUDPChannelStreamSession"(reference=w401, error in=w404, "MaxRate"=1000.0, "Multicast"=TRUE, "ClientPort"=u16 0, "ByteOrder"=w386) -> (reference out=w403:T6, error out=w402:errorcluster)
        n122 = Array Size(array=w378) -> (size(s)=w399:i32)
        n123 = Initialize Array(w400, w399) -> (w392:waveform(dbl)[])
        n124 = property on="Chart" class="WFChart (strict)"("History Data"=waveform(dbl)[][] []) -> ()  [unwired: 2 in, 2 out]
        n125 = call <vilib>:"NI VeriStand - Deploy UDP Channel Streaming Session.vi"("error in (no error)"=w402, "UDPChannelStreamSession in"=w403) -> ("error out"=w396:errorcluster, "Packet IDs"=w389:i32[], "Channel IDs"=w390:i32[], "UDPChannelStreamSession out"=w391:T6, "Max Packet Size"=w388:i32, "Port"=w397:u16, "UDP Multicast Address"=w395:string)  [unwired: 3 in]
        n126 = String To IP(1:w395) -> (0:w398:u32)
        n127 = call-poly <vilib>:"UDP Multicast Open.vi"("error in (no error)"=w396, "multicast addr"=w398, "port"=w397) -> ("error out"=w383:errorcluster, "connection ID"=w387:refnum<k16>)  [unwired: 6 in, 1 out]
        n128 = Bundle By Name(cluster=w393, "Initialized Waveform"=w392, "VS UDP Session"=w391, "Channel IDs"=w390, "Packet IDs"=w389, "Max Packet Size"=w388, "UDP Ref"=w387) -> (w385:T7)
        n129 = Select(t=UDP_Streaming_State."Stop Acq", s=w383, f=UDP_Streaming_State."Run" ("Action")) -> (s? t:f=w380:T4)
      }
      frame "Run" {
        n130 = Unbundle By Name(w411) -> ("Initialized Waveform"=w417:waveform(dbl)[], "Channel IDs"=w416:i32[], "Packet IDs"=w415:i32[], "UDP Ref"=w414:refnum<k16>, "Max Packet Size"=w413:i32)
        n131 = UDP Read(connection ID=w414, max size (548)=w413, timeout ms (25000)=2500, 8:w409) -> (data out=w419:string, error out=w420:errorcluster, 3:w421:refnum<k16>)  [unwired: 2 out]
        n132 = case shown="No Error" w420 {
          selector: w420 -> [w432 w478]
          tunnel: w415 -> [w427 _]
          tunnel: w419 -> [w430 _]
          tunnel: w416 -> [w429 _]
          tunnel: w417 -> [w428 _]
          tunnel: [w433 w476] -> w408
          tunnel: w421 -> [_ _]
          tunnel: w407 -> [w423 _]
          tunnel: [w422 w477] -> w412
          tunnel: w411 -> [w422 w477]
          frame No Error {
            n133 = Unflatten From String(type=T17 {"ID"=0, "t0"=0.0, "dt"=0.0, "Channel IDs"=[], "Channel Data"=[], "Sample Offset"=0} ("UDP Data Packet"), binary string=w430, byte order (0:big-endian, network order)=w423, error in (no error)=w432) -> (value=w424:T17, error out=w433:errorcluster)  [unwired: 1 in, 1 out]
            n134 = Unbundle By Name(w424) -> ("ID"=w425:i32)
            n135 = Search 1D Array(1D array=w427, element=w425) -> (index of element=w426:i32)  [unwired: 1 in]
            n136 = case shown="Default" w426 {
              tunnel: w429 -> [_ w445]
              tunnel: w428 -> [_ w444]
              tunnel: w427 -> [_ w442]
              tunnel: w424 -> [_ w441]
              frame -1 {
                # "This is a packet from a different UDP session. Ignore it."
              }
              frame Default {
                n137 = Unbundle By Name(w441) -> ("ID"=w440:i32, "Channel IDs"=w439:i32[], "Channel Data"=w438:dbl[][], "t0"=w437:dbl, "dt"=w436:dbl)  [unwired: 1 out]
                n138 = To Time Stamp(1:w437) -> (0:w443:timestamp)
                n139 = for {
                  tunnel: w445 -> [w458] mode=indexing
                  tunnel: w442 -> [w460] mode=indexing
                  tunnel: w440 -> [w459]
                  tunnel: w438 -> [w452]
                  tunnel: w439 -> [w451]
                  shift-right: [w447] -> w435
                  shift-left: w444 -> [w450]
                  tunnel: w443 -> [w449]
                  tunnel: w436 -> [w448]
                  i -> [w453]
                  n140 = Search 1D Array(1D array=w451, element=w458) -> (index of element=w454:i32)  [unwired: 1 in]
                  n141 = Equal?(x=w460, y=w459) -> (x = y?=w457:bool)
                  n142 = Greater Or Equal To 0?(x=w454) -> (x >= 0?=w456:bool)
                  n143 = Compound Arithmetic op=AND(w457, w456) -> (w455:bool)
                  n144 = case shown="True" w455 {
                    tunnel: w454 -> [_ w466]
                    tunnel: w453 -> [_ w462]
                    tunnel: w452 -> [_ w467]
                    tunnel: w450 -> [w461 w468]
                    tunnel: w449 -> [_ w465]
                    tunnel: w448 -> [_ w464]
                    tunnel: [w461 w463] -> w447
                    frame False {
                      # "This channel is not in this UDP Data Packet."
                    }
                    frame True {
                      n145 = in-place {
                        in-place-border: w467 -> [w474]
                        in-place-border: w466 -> [w473]
                        in-place-border: w465 -> [w471]
                        in-place-border: w464 -> [w470]
                        n146 = in-place-array #1(w468, w462) -> (w475:waveform(dbl))
                        n147 = Index Array(array=w474, index (row)=w473) -> (element=w472:dbl[])  [unwired: 1 in]
                        n148 = Bundle By Name(cluster=w475, "Y"=w472, "t0"=w471, "dt"=w470) -> (w469:waveform(dbl))
                        n149 = in-place-array #1(w469) -> (w463:waveform(dbl)[])  [unwired: 1 out]
                      }
                    }
                  }
                }
                n150 = case shown="False" "Hold" {
                  tunnel: w435 -> [w446 _]
                  frame False {
                    "Chart" <- w446
                  }
                  frame True {
                  }
                }
              }
            }
          }
          frame Error {
            # "Error 113 can be returned if you read a UDP packet from another stream session that is larger than the max number of bytes expected for the packets in your stream session. Ignore this error."
            n151 = call <vilib>:"Clear Errors.vi"("error in (no error)"=w478) -> ("error out"=w476:errorcluster)  [unwired: 6 in]
          }
        }
      }
      frame "Stop Acq" {
        n152 = case shown="\"Start Acq\", \"Run\"" w480 {
          tunnel: w484 -> [_ w485]
          frame Default {
          }
          frame "Start Acq", "Run" {
            n153 = Unbundle By Name(w485) -> ("VS UDP Session"=w486:T6, "UDP Ref"=w487:refnum<k16>)
            n154 = flat-sequence {
              tunnel: w487 -> [w490]
              tunnel: w486 -> [w489]
              tunnel: [w488] -> _
              frame #0 {
                n155 = UDP Close(connection ID=w490) -> (error out=w493:errorcluster)  [unwired: 1 in, 1 out]
                n156 = call <vilib>:"NI VeriStand - Undeploy UDP Channel Streaming Session.vi"("error in (no error)"=w493, "UDPChannelStreamSession in"=w489) -> ("error out"=w491:errorcluster, "UDPChannelStreamSession out"=w492:T6)  [unwired: 8 in]
                n157 = call <vilib>:"NI VeriStand - Close UDP Channel Streaming Session.vi"("error in (no error)"=w491, "UDPChannelStreamSession in"=w492) -> ("error out"=w488:errorcluster)  [unwired: 9 in]
              }
            }
          }
        }
        n158 = property on="Chart" class="WFChart (strict)"("History Data"=waveform(dbl)[][] []) -> ()  [unwired: 2 in, 2 out]
        n159 = call <vilib>:"Simple Error Handler.vi"("error in (no error)"=w482) -> ()  [unwired: 4 in, 5 out]
        n160 = call <vilib>:"Clear Errors.vi"("error in (no error)"=w482) -> ("error out"=w481:errorcluster)  [unwired: 6 in]
      }
      frame "Exit" {
      }
    }
  }
  n161 = Unregister For Events(event registration refnum=w17) -> (error out=w32:errorcluster)  [unwired: 1 in]
  n162 = flat-sequence {
    tunnel: w34 -> [_]
    tunnel: w32 -> [w501]
    tunnel: w10 -> [w502]
    tunnel: w28 -> [w499]
    tunnel: w21 -> [w498]
    frame #0 {
      n163 = call <vilib>:"NI VeriStand - Close Engine State Change Notification.vi"("SystemStateRefs"=w498) -> ()  [unwired: 10 in, 1 out]
      n164 = Destroy User Event(user event=w502, error in=w501) -> (error out=w500:errorcluster)
      n165 = Destroy User Event(user event=w499, error in=w500) -> ()  [unwired: 1 out]
    }
  }
